vi "Receive Control Mouse Down Event.vi"(8 "error in (no error)":errorcluster, 10 "ControlMouseDownMsg":refnum<class "ControlMouseDownMsg.lvclass">, 11 "File Explorer In":refnum<class "File Explorer.lvclass">) -> (0 "error out":errorcluster, 3 "File Explorer Out":refnum<class "File Explorer.lvclass">)   [LabVIEW 2020, in "File Explorer.lvlib" / "File Explorer.lvclass"]
doc: "<License>\nCopyright © 2017 Composed Systems, LLC | All rights reserved\nwww.composed.io\n\nAuthor: Ethan Stern <ethan.stern@composed.io>\n\nThis software is provided \"AS IS\" WITHOUT WARRANTIES, either express or implied, AND IS FOR EDUCATIONAL PURPOSES ONLY.\n</License>"
uses:
  <vilib>/gpm_packages/@cs/file-explorer-extension/Source/File Explorer/File Explorer/File Explorer.lvclass
  <vilib>/gpm_packages/@cs/mva-viewable/Source/ActorEvents/IEventAggregator Messages/ControlMouseDownMsg/ControlMouseDownMsg.lvclass
  <vilib>/gpm_packages/@cs/mva-viewable/Source/ActorEvents/IEventAggregator Messages/ControlMouseDownMsg/ControlMouseDownMsg.lvclass/ControlMouseDownMsg.ctl
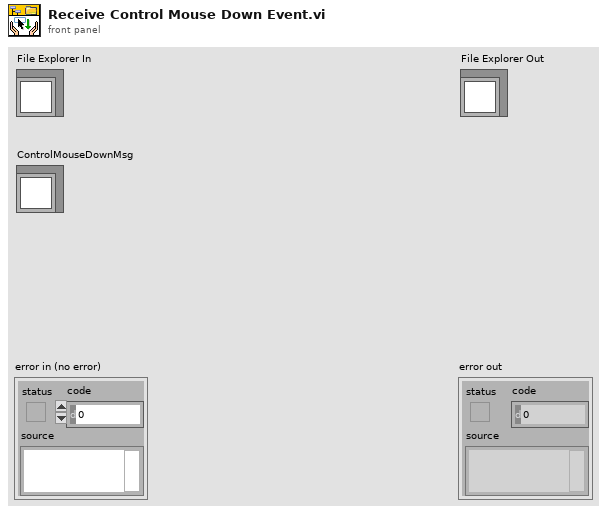
[diagram p1: front panel]
types:
  T1 = typedef "LVPoint32TypeDef.ctl" = cluster{"Horizontal":i32, "Vertical":i32}
  T2 = cluster{"Shift":bool, "Ctrl":bool, "Alt":bool, "Cmd":bool, "Opt":bool}
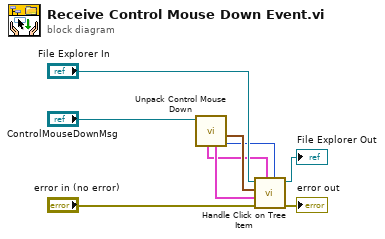
[diagram p0: block diagram]
diagram:
  n1 = call <vilib>:"Unpack Control Mouse Down.vi"("ControlMouseDownMsg"="ControlMouseDownMsg") -> ("Button"=w1:u16, "Coords"=w6:T1, "Mods"=w3:cluster{"Double Click":bool, "Menu Key":bool}, "PlatMods"=w2:T2)  [unwired: 4 in, 3 out]
  n2 = call-dynamic "Handle Click on Tree Item.vi"("Button"=w1, "PlatMods"=w2, "error in (no error)"="error in (no error)", "Mods"=w3, "Coords"=w6, "File Explorer in"="File Explorer In") -> ("error out"=→"error out":errorcluster, "File Explorer out"=→"File Explorer Out":refnum<class "File Explorer.lvclass">)  [unwired: 4 in]
